vi "Optics.vi"(8 "error in (no error)":errorcluster, 10 "Optics POST Input Cluster":T1, 11 "Controls and Indicators\nReferences":T3) -> (0 "error out":errorcluster, 2 "Diagnostics Image_Diagnostics":T2(plugin-control))   [LabVIEW 2019, in "ZenGage v3.0 UI.lvclass"]
uses:
  ZenGage v3.0 UI.lvclass
  Type Definitions/Controls and Indicators/Select a part (combobox).ctl
  Type Definitions/Controls and Indicators/EDL control references.ctl
  Type Definitions/Controls and Indicators/Diagnostics control referencs.ctl
  Type Definitions/Controls and Indicators/Inspection control references.ctl
  Type Definitions/Controls and Indicators/General_Control references.ctl
  Type Definitions/Controls and Indicators/Controls and Indicators Cluster.ctl
  Type Definitions/Diagnostics/OpticsPOSTInputCluster.ctl
  Type Definitions/General/Master sample references.ctl
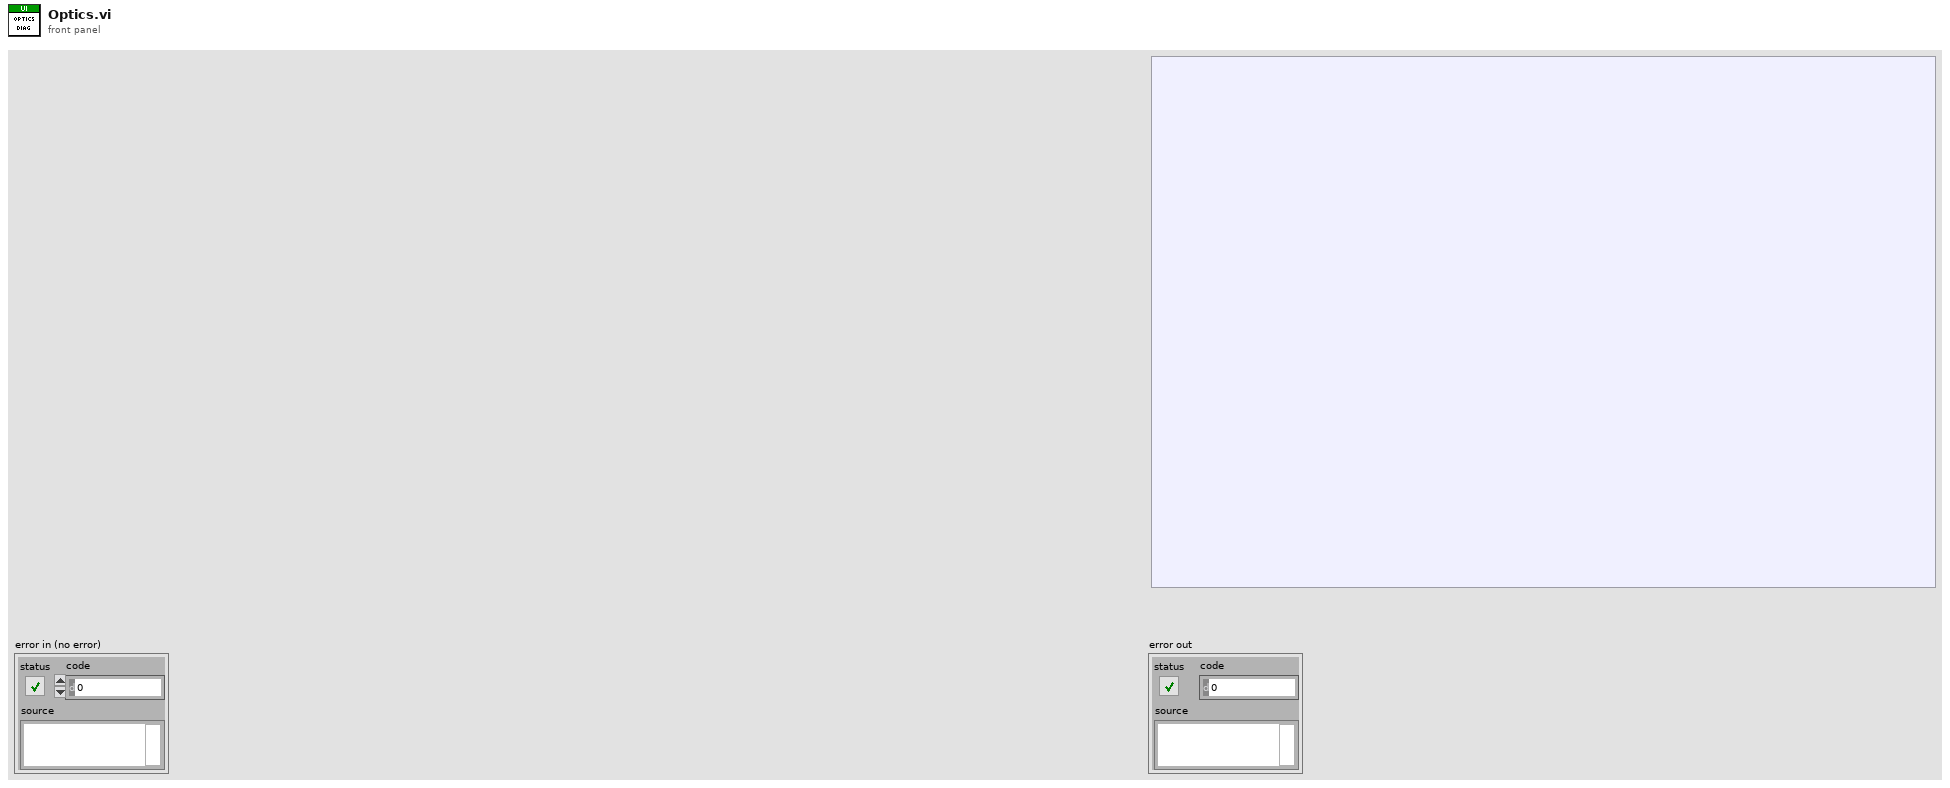
[diagram p1: front panel]
types:
  T1 = typedef "ZenGage v3.0 UI.lvclass/OpticsPOSTInputCluster.ctl" = cluster{"Dust Percentage":dbl, "Diagnostics Sstatus string":string, "Pass?":bool, "final image":T2}
  T2 = typedef "IMAQ Image.ctl" = refnum<image>
  T3 = typedef "ZenGage v3.0 UI.lvclass/Controls and Indicators Cluster.ctl" = cluster{"General":T4, "Inspection":T5, "Diagnostics":T6, "Edit Tolerance Limits":T7, "Master sample":T8}
  T4 = typedef "ZenGage v3.0 UI.lvclass/General_Control references.ctl" = cluster{"Main Tab":refnum<vi>, "Inspection SubPanel_Inspection":refnum<vi>, "Zen Logo_Inspection":refnum<vi>, "SoftwareExit":refnum<vi>, "Loading Bar VI Ref":refnum<vi>, "Right Pane Tab":refnum<vi>, "Image Reference array":refnum<vi>[], "Command tab":refnum<vi>, "Inspection subTab control ref":refnum<vi>, "SelectionCluster":cluster{"ok":refnum<vi>, "confirm":refnum<vi>, "reset":refnum<vi>, "change":refnum<vi>, "TOTAL COUNT":refnum<vi>, "REEL COUNT":refnum<vi>, "PART NAME":refnum<vi>, "VERIFIED":refnum<vi>, "OPERATOR NAME":refnum<vi>, "Select message":refnum<vi>}, "Event  Reason  List":refnum<vi>, "Event reason blink":refnum<vi>, "Event reason switching tab":refnum<vi>, "confirm_eventReason":refnum<vi>}
  T5 = typedef "ZenGage v3.0 UI.lvclass/Inspection control references.ctl" = cluster{"Inspection Status":refnum<vi>, "Run_Inspection":refnum<vi>, "Pause_Inspection":refnum<vi>, "Stop_Inspection":refnum<vi>, "Settings_Inspection":refnum<vi>, "Inspection Images VI Ref":refnum<vi>, "Pass-Fail Indicator String":refnum<vi>, "Analytics_Inspection":refnum<vi>, "Label array":refnum<vi>[], "Analytics VI\nreference":refnum<vi>, "Counts":refnum<vi>, "Cards array":refnum<vi>, "Counts array":refnum<vi>[]}
  T6 = typedef "ZenGage v3.0 UI.lvclass/Diagnostics control referencs.ctl" = cluster{"Diagnostics Tab":refnum<vi>, "Dust indicator :":refnum<vi>, "Logout_Diagnostics":refnum<vi>, "CAMERA STATUS MESSAGE":refnum<vi>, "BUZZER OFF":refnum<vi>, "PAUSE":refnum<vi>, "STOP":refnum<vi>, "RUN":refnum<vi>, "Current Diagnostics Status":refnum<vi>, "Select a diagnostics":refnum<vi>, "Diagnostics Status":refnum<vi>, "Select a sub diagnostics":refnum<vi>, "Optics img":refnum<vi>, "Diagnostics Status\nString":refnum<vi>}
  T7 = typedef "ZenGage v3.0 UI.lvclass/EDL control references.ctl" = cluster{"Tolerance Limits Listbox":refnum<vi>, "Enable Disable":refnum<vi>, "Cluster of limits":refnum<vi>, "Thresholds limits":refnum<vi>, "Update List":refnum<vi>, "Save":refnum<vi>, "Back_Edit Tolerance":refnum<vi>, "logout":refnum<vi>, "Select a part":refnum<vi>, "Bias Correction":refnum<vi>, "Linearity Correction":refnum<vi>, "Select a Rack":refnum<vi>, "ETS tab":refnum<vi>, "Factory reset":refnum<vi>, "Door\nPoka Yoke":refnum<vi>, "Fail count reverse":refnum<vi>, "ETL count error message":refnum<vi>, "ETL help string":refnum<vi>}
  T8 = typedef "Master sample references.ctl" = cluster{"Master sample message":refnum<vi>, "Master sample tab":refnum<vi>, "Next":refnum<vi>, "Repeat":refnum<vi>, "Master sample part message":refnum<vi>}
  T9 = enum32{"Arduino Motor", "Sensor trigger", "Hardware Button", "Camera Optics"}
  T10 = enum32{"Invalid", "Standard", "Closed", "Hidden", "Minimized", "Maximized"}
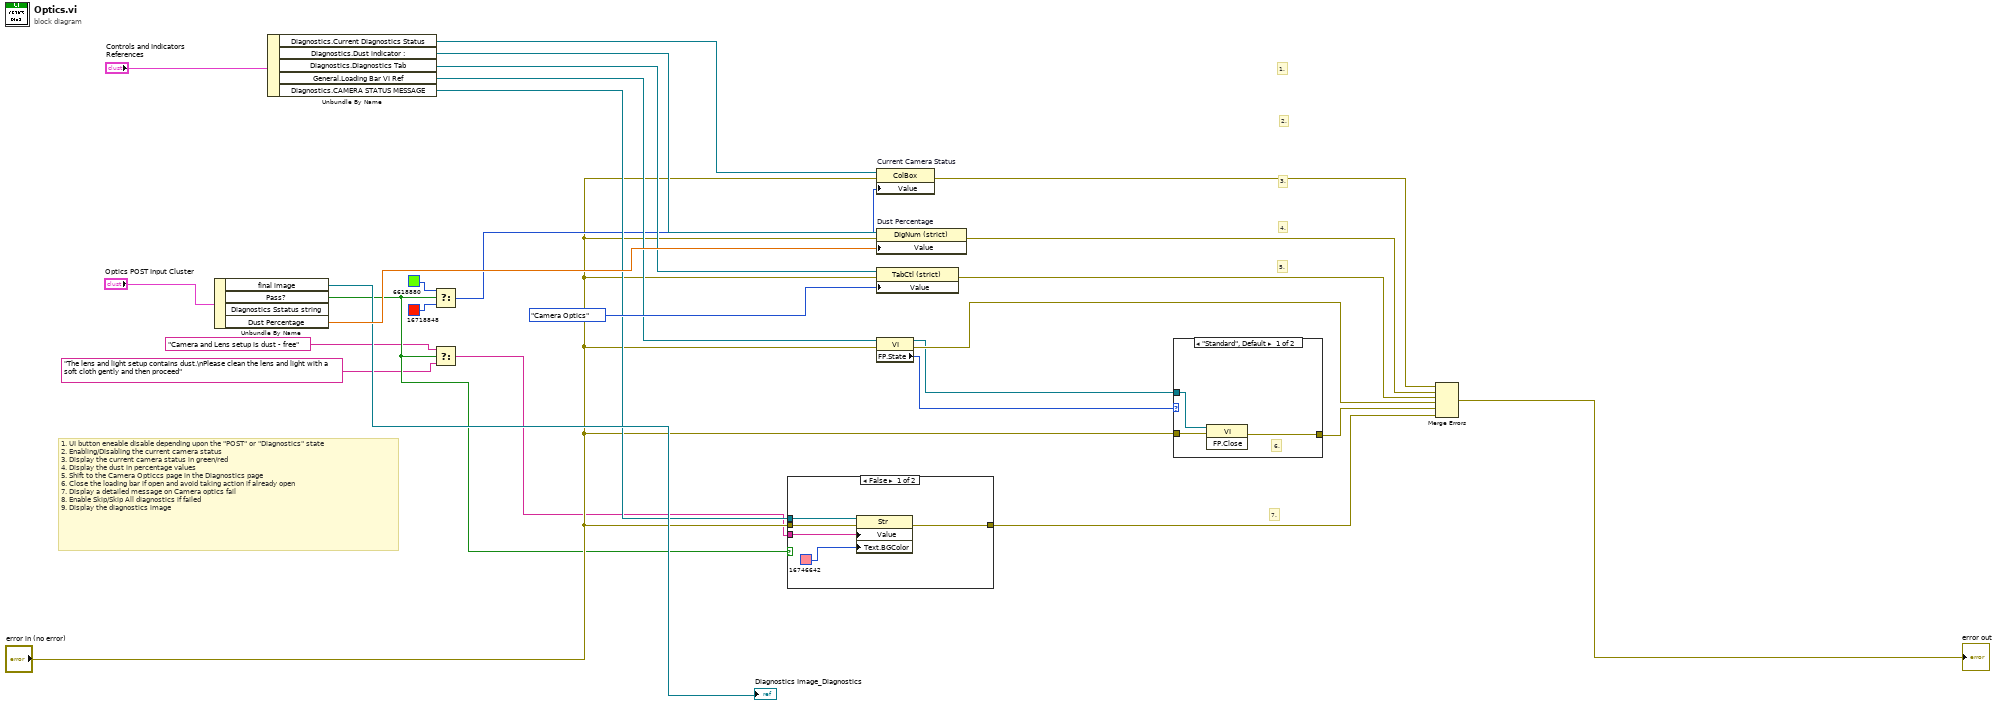
[diagram p0: block diagram]
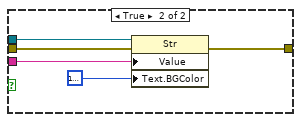
[diagram p2: hidden frame]
diagram:
  # "1."
  # "7."
  # "5."
  # "4."
  # "3."
  # "2."
  # "1. UI button eneable disable depending upon the \"POST\" or \"Diagnostics\" state\n2. Enabling/Disabling the current camera status\n3. Display the current camera status in green/red\n4. Display the dust in percentage values\n5. Shift to the Camera Opticcs page in the Diagnostics page\n6. Close the loading bar if open and avoid taking action if already open\n7. Display a detailed message on Camera optics fail\n8. Enable Skip/Skip All diagnostics if failed\n9. Display the diagnostics image"
  n1 = Unbundle By Name("Optics POST Input Cluster") -> ("final image"=→"Diagnostics Image_Diagnostics":T2, "Pass?"=w4:bool, "Dust Percentage"=w27:dbl)  [unwired: 1 out]
  n2 = Unbundle By Name("Controls and Indicators\nReferences") -> ("Diagnostics.Current Diagnostics Status"=w11:refnum<vi>, "Diagnostics.Dust indicator :"=w12:refnum<vi>, "Diagnostics.Diagnostics Tab"=w13:refnum<vi>, "General.Loading Bar VI Ref"=w14:refnum<vi>, "Diagnostics.CAMERA STATUS MESSAGE"=w15:refnum<vi>)
  n3 = Select(t=u32 6618880, s=w4, f=u32 16718848) -> (s? t:f=w8:u32)
  n4 = Select(t="Camera and Lens setup is dust - free", s=w4, f="The lens and light setup contains dust.\nPlease clean the lens and light with a soft cloth gently and then proceed") -> (s? t:f=w1:string)
  n5 = case shown="False" w4 {
    tunnel: w15 -> [w29 w36]
    tunnel: w1 -> [w28 w37]
    tunnel: "error in (no error)" -> [w32 w34]
    tunnel: [w31 w33] -> w23
    frame False {
      n6 = property class="Str"(reference=w29, error in=w32, "Value"=w28, "Text.BGColor"=u32 16746642) -> (error out=w31:errorcluster)  [unwired: 1 out]
    }
    frame True {
      n7 = property class="Str"(reference=w36, error in=w34, "Value"=w37, "Text.BGColor"=u32 16777216) -> (error out=w33:errorcluster)  [unwired: 1 out]
    }
  }
  n8 = property on="Current Camera Status" class="ColBox"(reference=w11, error in="error in (no error)", "Value"=w8) -> (error out=w19:errorcluster)  [unwired: 1 out]
  n9 = property on="Dust Percentage" class="DigNum (strict)"(reference=w12, error in="error in (no error)", "Value"=w27) -> (error out=w20:errorcluster)  [unwired: 1 out]
  n10 = property class="TabCtl (strict)"(reference=w13, error in="error in (no error)", "Value"=T9."Camera Optics") -> (error out=w24:errorcluster)  [unwired: 1 out]
  n11 = property class="VI"(reference=w14, error in="error in (no error)") -> (reference out=w18:refnum<vi>, error out=w21:errorcluster, "FP.State"=w17:T10)
  n12 = case shown="\"Standard\", Default" w17 {
    tunnel: "error in (no error)" -> [w40 w41]
    tunnel: [w39 w41] -> w22
    tunnel: w18 -> [w38 _]
    frame "Standard", Default {
      # "6."
      n13 = invoke class="VI" method="FP.Close"() -> ()  [unwired: 3 in, 3 out]
      n14 = invoke class="VI" method="FP.Close"(reference=w38, error in=w40) -> (error out=w39:errorcluster)  [unwired: 1 in, 2 out]
    }
    frame "Closed" {
    }
  }
  n15 = Merge Errors(w19, w20, w24, w21, w22, w23) -> (→"error out":errorcluster)
